vi "UserEncoder.vi"(0 "RS n":i32, 2 "Refnum in":T1, 5 "RS k":i32, 9 "Const. length":i32, 11 "error in (no error)":errorcluster, 13 "Tab Control in":enum32{"No coding", "RS only", "RS+Conv."}(ring)) -> (4 "Encoded bitstream":i8[](array[numeric]), 6 "Information bits":i8[](array[numeric]), 8 "Refnum out":T1, 15 "error out":errorcluster)   [LabVIEW 2012]
uses:
  <vilib>/addons/Modulation/Digital/Support/Controls/MT Generic Refnum.ctl
  <vilib>/addons/Modulation/Digital/General/MT Generate Bits (Galois, PN Order).vi
  <vilib>/addons/Modulation/Digital/Channel Coding/MT RS Symbol Encoder (normal).vi
  <vilib>/addons/Modulation/Digital/Channel Coding/MT Convolutional Encoder (Rate).vi
  <vilib>/addons/Modulation/niDMT.lvlib
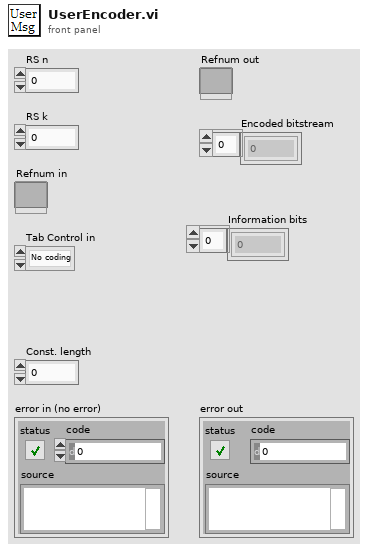
[diagram p1: front panel]
types:
  T1 = typedef "niDMT.lvlib/MT Generic Refnum.ctl" = refnum<k20>
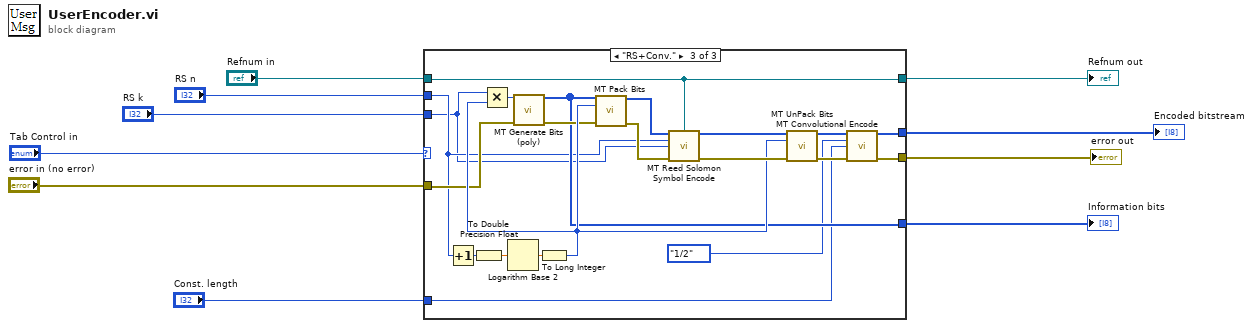
[diagram p0: block diagram]
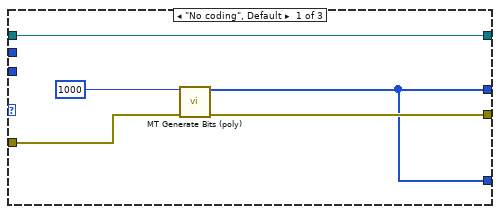
[diagram p2: hidden frame]
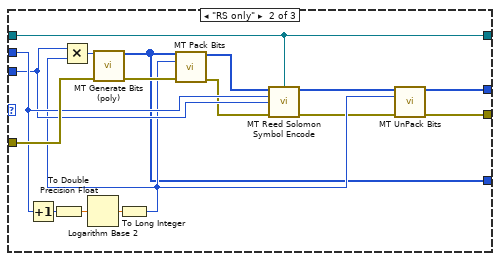
[diagram p3: hidden frame]
diagram:
  n1 = case shown="\"RS+Conv.\"" "Tab Control in" {
    tunnel: [w11 w19 w35] -> w3
    tunnel: "RS n" -> [_ w25 w40]
    tunnel: "RS k" -> [_ w24 w39]
    tunnel: "error in (no error)" -> [w13 w27 w42]
    tunnel: "Refnum in" -> [w14 w18 w41]
    tunnel: "Const. length" -> [_ _ w33]
    tunnel: [w14 w18 w41] -> w9
    tunnel: [w12 w17 w36] -> w10
    tunnel: [w11 w16 w43] -> w1
    frame "No coding", Default {
      n2 = call-poly <vilib>:"MT Generate Bits (poly).vi"("total bits (128)"=1000, "error in (no error)"=w13) -> ("output bit stream"=w11:i8[], "error out"=w12:errorcluster)  [unwired: 11 in, 1 out]
    }
    frame "RS only" {
      n3 = Increment(x=w25) -> (x+1=w31:i32)
      n4 = To Double Precision Float(number=w31) -> (double precision float=w32:dbl)
      n5 = Logarithm Base 2(1:w32) -> (0:w30:dbl)
      n6 = To Long Integer(number=w30) -> (32bit integer=w21:i32)
      n7 = Multiply(x=w24, y=w21) -> (x*y=w29:i32)
      n8 = call-poly <vilib>:"MT Generate Bits (poly).vi"("total bits (128)"=w29, "error in (no error)"=w27) -> ("output bit stream"=w16:i8[], "error out"=w28:errorcluster)  [unwired: 11 in, 1 out]
      n9 = call <vilib>:"MT Pack Bits.vi"("input bit stream"=w16, "bits per integer"=w21, "error in (no error)"=w28) -> ("output integers"=w26:i32[], "error out"=w23:errorcluster)  [unwired: 11 in]
      n10 = call-poly <vilib>:"MT Reed Solomon Symbol Encode.vi"("input symbols"=w26, "modulation session"=w18, "code word length (n), symbols"=w25, "data word length (k), symbols"=w24, "error in (no error)"=w23) -> ("output symbols"=w22:i32[], "error out"=w20:errorcluster)  [unwired: 9 in]
      n11 = call <vilib>:"MT UnPack Bits.vi"("input integers"=w22, "bits per integer"=w21, "error in (no error)"=w20) -> ("output bit stream"=w19:i8[], "error out"=w17:errorcluster)  [unwired: 11 in]
    }
    frame "RS+Conv." {
      n12 = Increment(x=w40) -> (x+1=w45:i32)
      n13 = To Double Precision Float(number=w45) -> (double precision float=w44:dbl)
      n14 = Logarithm Base 2(1:w44) -> (0:w46:dbl)
      n15 = To Long Integer(number=w46) -> (32bit integer=w52:i32)
      n16 = Multiply(x=w39, y=w52) -> (x*y=w47:i32)
      n17 = call-poly <vilib>:"MT Generate Bits (poly).vi"("total bits (128)"=w47, "error in (no error)"=w42) -> ("output bit stream"=w43:i8[], "error out"=w48:errorcluster)  [unwired: 11 in, 1 out]
      n18 = call <vilib>:"MT Pack Bits.vi"("input bit stream"=w43, "bits per integer"=w52, "error in (no error)"=w48) -> ("output integers"=w49:i32[], "error out"=w50:errorcluster)  [unwired: 11 in]
      n19 = call-poly <vilib>:"MT Reed Solomon Symbol Encode.vi"("input symbols"=w49, "modulation session"=w41, "code word length (n), symbols"=w40, "data word length (k), symbols"=w39, "error in (no error)"=w50) -> ("output symbols"=w51:i32[], "error out"=w53:errorcluster)  [unwired: 9 in]
      n20 = call <vilib>:"MT UnPack Bits.vi"("input integers"=w51, "bits per integer"=w52, "error in (no error)"=w53) -> ("output bit stream"=w38:i8[], "error out"=w37:errorcluster)  [unwired: 11 in]
      n21 = call-poly <vilib>:"MT Convolutional Encode.vi"("input bit stream"=w38, "rate (k/n)"=enum16{"1/2", "1/3", "1/4", "2/3", "3/4"}."1/2", "constraint length (K)"=w33, "error in (no error)"=w37) -> ("output bit stream"=w35:i8[], "error out"=w36:errorcluster)  [unwired: 9 in, 1 out]
    }
  }
  "error out" <- w10
  "Refnum out" <- w9
  "Encoded bitstream" <- w3
  "Information bits" <- w1
